vi "CloseSoundCard.vi"(3 "All Info":T1 {"Data Set"."Settings"."Time" format="%<%H:%M\n%d/%m/%y>T"; "task ID" format="%.0x"}) -> ()   [LabVIEW 2014]
uses:
  <userlib>/CurtinCode/AllDataCtrl.ctl
  <userlib>/CurtinCode/DataControl.ctl
  <userlib>/CurtinCode/SettingsControl.ctl
  <vilib>/sound2/lvsound2.llb/Sound Input Task ID.ctl
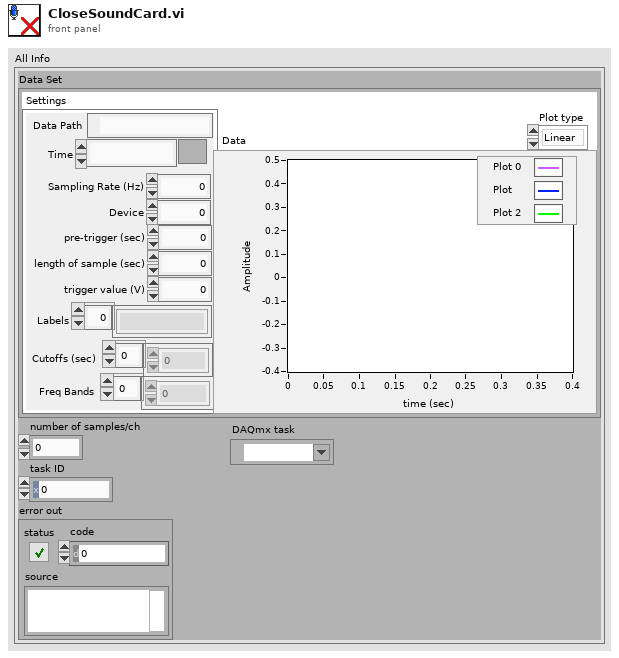
[diagram p1: front panel]
types:
  T1 = typedef "AllDataCtrl.ctl" = cluster{"Data Set":T2, "number of samples/ch":i32, "task ID":T4, "error out":errorcluster, "DAQmx task":refnum<k21>}
  T2 = typedef "DataControl.ctl" = cluster{"Settings":T3, "Data":cluster{i32, dbl, "data":dbl[]}[], "Plot type":enum16{"Linear", "log"}}
  T3 = typedef "SettingsControl.ctl" = cluster{"Data Path":path, "Time":timestamp, "Sampling Rate (Hz)":u16, "Device":u16, "pre-trigger (sec)":dbl, "length of sample (sec)":dbl, "trigger value (V)":dbl, "Labels":string[], "Cutoffs (sec)":dbl[], "Freq Bands":dbl[]}
  T4 = typedef "Sound Input Task ID.ctl" = u32
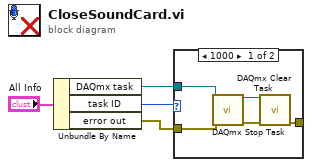
[diagram p0: block diagram]
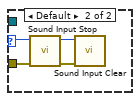
[diagram p2: hidden frame]
diagram:
  n1 = Unbundle By Name("All Info") -> ("DAQmx task"=w1:refnum<k21>, "task ID"=w2:T4, "error out"=w4:errorcluster)
  n2 = case shown="1000" w2 {
    selector: w2 -> [_ w10]
    tunnel: w4 -> [w7 w13]
    tunnel: w1 -> [w6 _]
    tunnel: [w5 _] -> _
    frame 1000 {
      n3 = call <vilib>:"DAQmx Stop Task.vi"("task/channels in"=w6, "error in"=w7) -> ("task out"=w9:refnum<k21>, "error out"=w8:errorcluster)  [unwired: 12 in]
      n4 = call <vilib>:"DAQmx Clear Task.vi"("task in"=w9, "error in"=w8) -> ("error out"=w5:errorcluster)  [unwired: 13 in]
    }
    frame Default {
      n5 = call <vilib>:"Sound Input Stop.vi"("error in (no error)"=w13, "task ID"=w10) -> ("error out"=w11:errorcluster, "task ID out"=w12:T4)  [unwired: 8 in]
      n6 = call <vilib>:"Sound Input Clear.vi"("error in (no error)"=w11, "task ID"=w12) -> ()  [unwired: 9 in, 1 out]
    }
  }
